vi "Write DAC Voltage - All DUTs - Single Channel.vi"(0 "Channel (0-5)":u32, 5 "Voltage":dbl format="%.3f V", 7 "Vref (-1: Unchanged)":dbl=-1.0 format="%.3f V", 11 "error in":errorcluster, 12 "Log (T)":bool=TRUE, 14 "FPGA":T1) -> (4 "Data Out":string[](array[string]), 15 "error out":errorcluster)   [LabVIEW 2017, in "Host SRL.lvlib"]
uses:
  Host SRL.lvlib
  Type Defs/WSVCAP SHL FPGA Enum.ctl
  Type Defs/WSVCAP SHL DUT Number Enum.ctl
panel:
  # "With all 6 devices selected in the Device Map:\n\nThis VI will write to 1 Channel, 1 DUT on Each Device (6 DUTs Total)\n\nFor example, a DUT value of any of the following: 1,5,9,13,17,21\nAll of them will be written to"
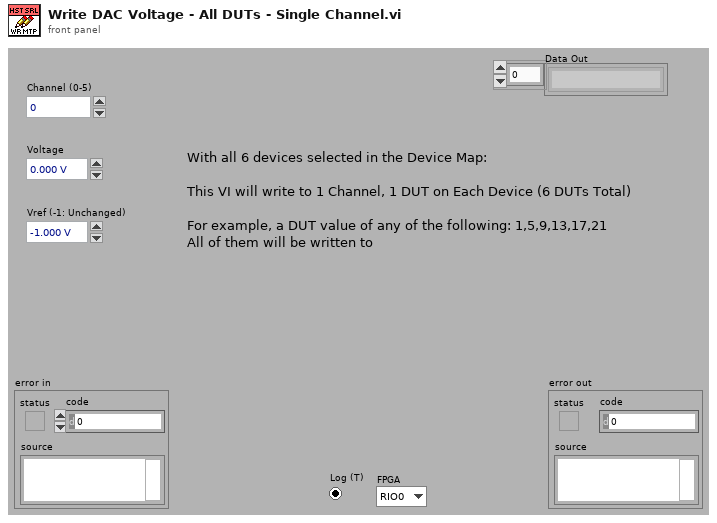
[diagram p1: front panel]
types:
  T1 = typedef "WSVCAP SHL FPGA Enum.ctl" = enum16{"RIO0", "RIO1"}
  T2 = typedef "WSVCAP SHL DUT Number Enum.ctl" = enum16{"DUT 01", "DUT 02", "DUT 03", "DUT 04", "DUT 05", "DUT 06", "DUT 07", "DUT 08", "DUT 09", "DUT 10", "DUT 11", "DUT 12", "DUT 13", "DUT 14", "DUT 15", "DUT 16", "DUT 17", "DUT 18", "DUT 19", "DUT 20", "DUT 21", "DUT 22", "DUT 23", "DUT 24"}
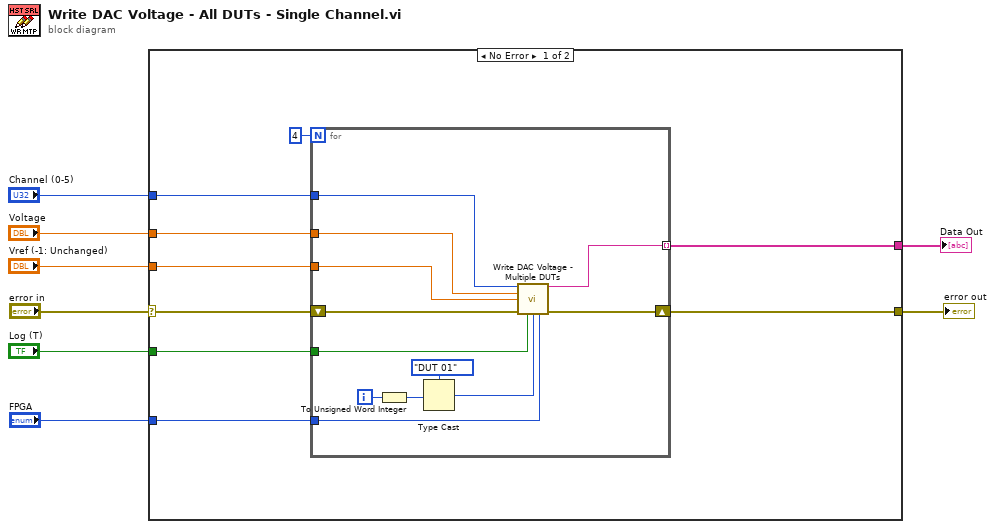
[diagram p0: block diagram]
diagram:
  n1 = case shown="No Error" "error in" {
    selector: "error in" -> [w14 _]
    tunnel: [w12 _] -> w8
    tunnel: "Log (T)" -> [w15 _]
    tunnel: "FPGA" -> [w16 _]
    tunnel: [w17 _] -> w4
    tunnel: "Channel (0-5)" -> [w10 _]
    tunnel: "Voltage" -> [w11 _]
    tunnel: "Vref (-1: Unchanged)" -> [w13 _]
    frame No Error {
      n2 = for {
        N: 4 -> [_]
        tunnel: [w24] -> w17 mode=indexing
        tunnel: w16 -> [w19]
        tunnel: w15 -> [w18]
        tunnel: w13 -> [w22]
        tunnel: w11 -> [w23]
        tunnel: w10 -> [w20]
        shift-right: [w25] -> w12
        shift-left: w14 -> [w26]
        i -> [w29]
        n3 = To Unsigned Word Integer(number=w29) -> (unsigned 16bit integer=w28:u16)
        n4 = Type Cast(type=WSVCAP_SHL_DUT_Number_Enum."DUT 01" ("DUT (Modulo 4)"), x=w28) -> (*(type *) &x=w21:T2)
        n5 = call "Write DAC Voltage - Multiple DUTs.vi"("Channel (0-5)"=w20, "Voltage"=w23, "Vref (-1: Unchanged)"=w22, "error in"=w26, "Log (T)"=w18, "DUT (Modulo 4)"=w21, "FPGA"=w19) -> ("Data Out"=w24:string, "error out"=w25:errorcluster)  [unwired: 7 in]
      }
    }
    frame Error {
    }
  }
  "error out" <- w8
  "Data Out" <- w4
